vi "Initialize Run Files and Variables.vi"(0 "Start TIme X":refnum<vi>, 2 "System Idle Pressure X":refnum<vi>, 3 "Reactor Number":i32, 5 "Header Connection txt Array":refnum<vi>, 7 "Queue Reactor X":refnum<vi>, 8 "Stop / Start Reactor X":refnum<vi>, 9 "Reactor Name":string, 10 "Username X":refnum<vi>, 11 "Save File Connection X":refnum<vi>, 12 "Experimental Details X":refnum<vi>, 14 "ALD Sequence for Reactor X":refnum<vi>, 15 "Save File JSON Connection X":refnum<vi>, 16 "GUID X":refnum<vi>, 19 "Logging Data X":refnum<vi>) -> ()   [LabVIEW 2021]
uses:
  <vilib>/Utility/error.llb/DialogType.ctl
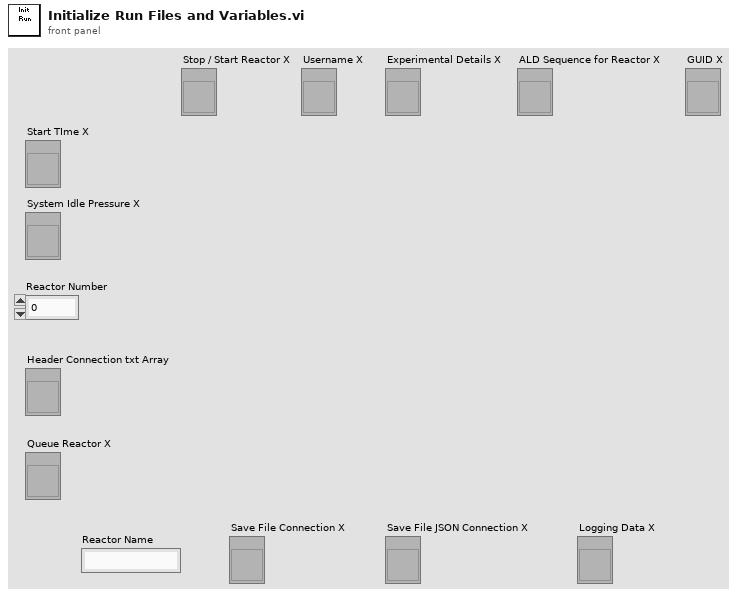
[diagram p1: front panel]
types:
  T1 = typedef "DialogType.ctl" = u16
  T2 = enum16{"open", "replace", "create", "open or create", "replace or create", "replace or create with confirmation"}
  T3 = cluster{"type":string, "meta":string, "payload":cluster{"GUID":string, "username":string, "experimentalDetails":string, "valveSequence":i32[][], "startTime":string, "reactorName":string}}
  T4 = cluster{"GUID":string, "username":string, "experimentalDetails":string, "valveSequence":i32[][], "startTime":string, "reactorName":string}
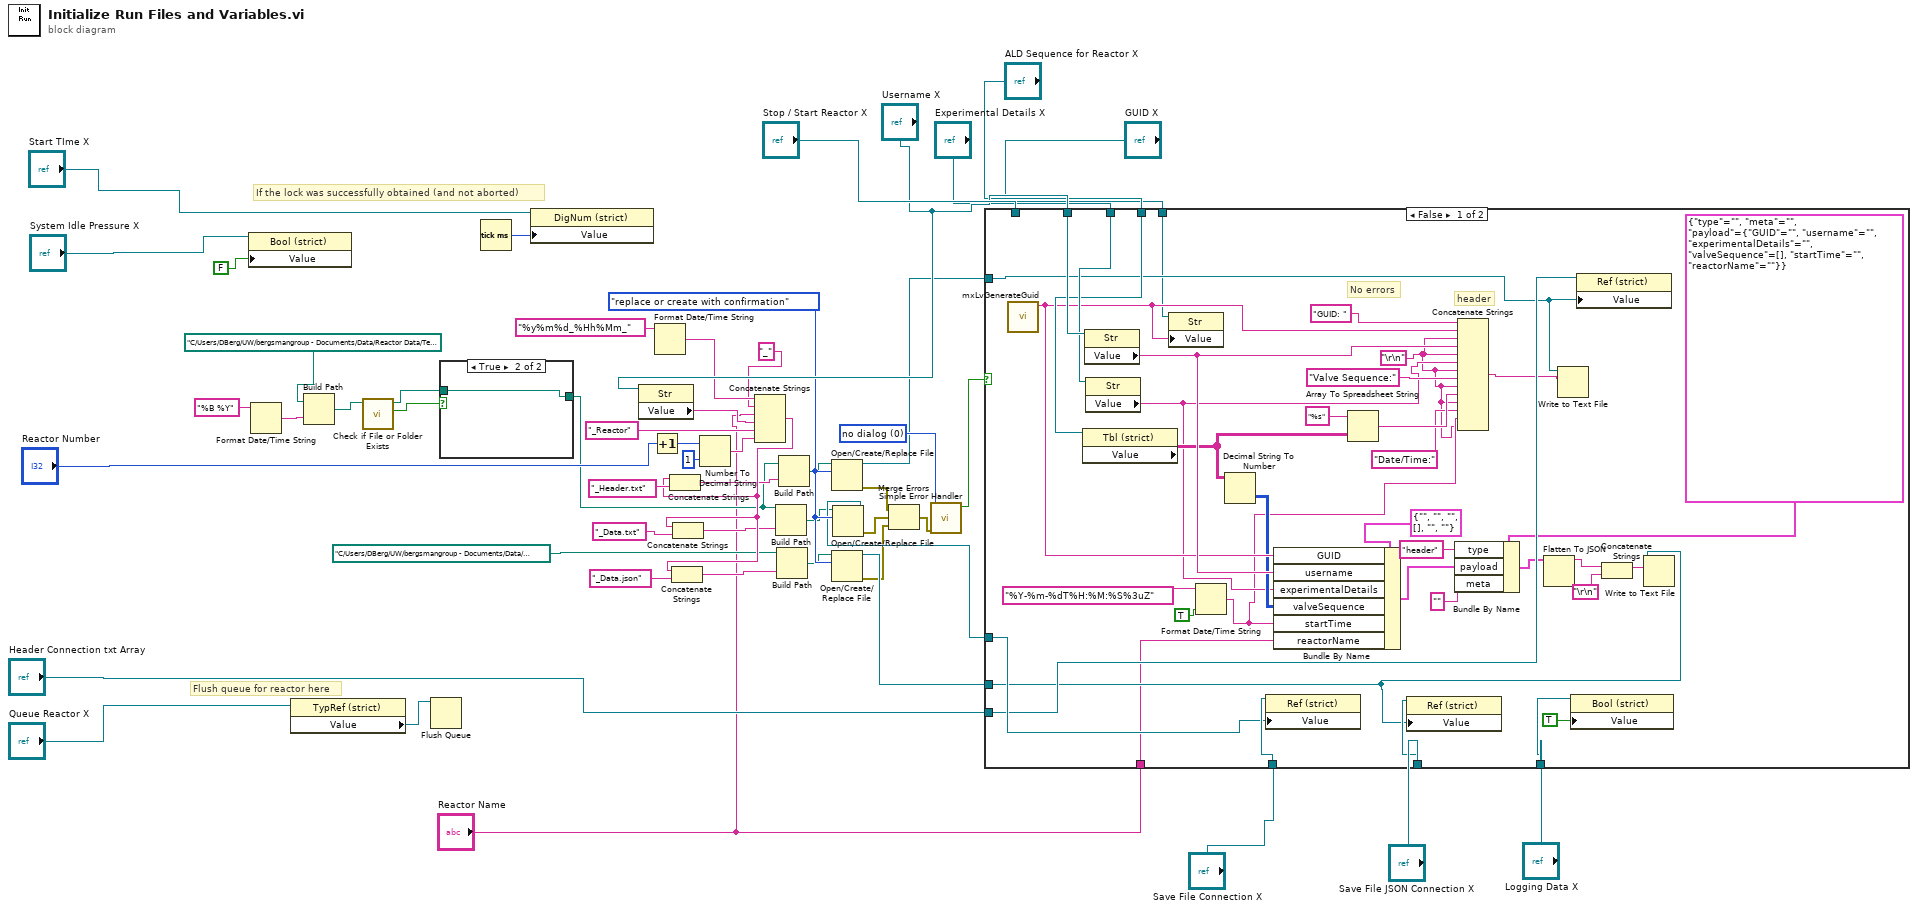
[diagram p0: block diagram]
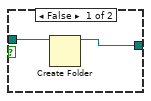
[diagram p2: hidden frame]
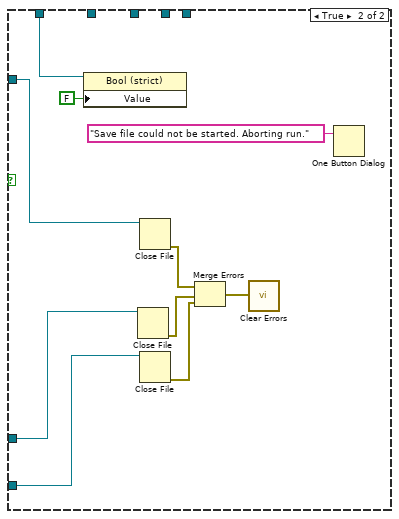
[diagram p3: hidden frame]
diagram:
  w31 = T1 0 items=["no dialog", "OK message", "continue or stop message", "OK message + warnings", "continue/stop + warnings"] ("type of dialog (OK msg:1)")
  w27 = T2."replace or create with confirmation" ("operation (0:open)")
  # "Flush queue for reactor here"
  # "If the lock was successfully obtained (and not aborted)"
  n1 = property class="Bool (strict)"(reference="System Idle Pressure X", "Value"=FALSE) -> ()  [unwired: 1 in, 2 out]
  n2 = Format Date/Time String(time format string (%c)="%B %Y") -> (date/time string=w9:string)  [unwired: 2 in]
  n3 = property class="TypRef (strict)"(reference="Queue Reactor X") -> ("Value"=w23:refnum<queue>)  [unwired: 1 in, 2 out]
  n4 = Build Path(base path=path "C:/Users/DBerg/UW/bergsmangroup - Documents/Data/Reactor Data/Text Files", name or relative path=w9) -> (appended path=w8:path)
  n5 = call <vilib>:"Check if File or Folder Exists.vi"("path"=w8) -> ("file or folder exists?"=w7:bool, "dup path"=w6:path)  [unwired: 8 in, 1 out]
  n6 = Flush Queue(queue=w23) -> ()  [unwired: 1 in, 3 out]
  n7 = case shown="True" w7 {
    tunnel: [w55 w56] -> w5
    tunnel: w6 -> [w54 w56]
    frame False {
      n8 = Create Folder(path (use dialog)=w54) -> (created path=w55:path)  [unwired: 2 in, 2 out]
    }
    frame True {
    }
  }
  n9 = Tick Count (ms)() -> (millisecond timer value=w36:u32)
  n10 = property class="DigNum (strict)"(reference="Start TIme X", "Value"=w36) -> ()  [unwired: 1 in, 2 out]
  n11 = property class="Str"(reference="Username X") -> ("Value"=w18:string)  [unwired: 1 in, 2 out]
  n12 = Increment(x="Reactor Number") -> (x+1=w37:i32)
  n13 = Format Date/Time String(time format string (%c)="%y%m%d_%Hh%Mm_") -> (date/time string=w3:string)  [unwired: 2 in]
  n14 = Number To Decimal String(number=w37, width (-)=i16 1) -> (decimal integer string=w19:string)
  n15 = Concatenate Strings(w3, "_" ("string"), "Reactor Name", w18, "_Reactor" ("string"), w19) -> (w29:string)
  n16 = Concatenate Strings(w29, "_Header.txt" ("string")) -> (w17:string)
  n17 = Concatenate Strings(w29, "_Data.json" ("string")) -> (w15:string)
  n18 = Concatenate Strings(w29, "_Data.txt" ("string")) -> (w16:string)
  n19 = Build Path(base path=w5, name or relative path=w16) -> (appended path=w13:path)
  n20 = Build Path(base path=path "C:/Users/DBerg/UW/bergsmangroup - Documents/Data/Reactor Data/JSON Files", name or relative path=w15) -> (appended path=w14:path)
  n21 = Build Path(base path=w5, name or relative path=w17) -> (appended path=w12:path)
  n22 = Open/Create/Replace File(file path (use dialog)=w12, operation (0:open)=w27) -> (refnum out=w25:refnum<file>, error out=w33:errorcluster)  [unwired: 4 in, 1 out]
  n23 = Open/Create/Replace File(file path (use dialog)=w14, operation (0:open)=w27) -> (refnum out=w24:refnum<file>, error out=w21:errorcluster)  [unwired: 4 in, 1 out]
  n24 = Open/Create/Replace File(file path (use dialog)=w13, operation (0:open)=w27) -> (refnum out=w26:refnum<file>, error out=w22:errorcluster)  [unwired: 4 in, 1 out]
  n25 = Merge Errors(w33, w22, w21) -> (w32:errorcluster)
  n26 = call <vilib>:"Simple Error Handler.vi"("type of dialog (OK msg:1)"=w31, "error in (no error)"=w32) -> ("error?"=w30:bool)  [unwired: 3 in, 4 out]
  n27 = case shown="False" w30 {
    tunnel: "Logging Data X" -> [w93 _]
    tunnel: "Stop / Start Reactor X" -> [_ w103]
    tunnel: "Username X" -> [w91 _]
    tunnel: "Experimental Details X" -> [w90 _]
    tunnel: "ALD Sequence for Reactor X" -> [w89 _]
    tunnel: "Save File Connection X" -> [w86 _]
    tunnel: w26 -> [w85 w99]
    tunnel: w25 -> [w80 w100]
    tunnel: "Save File JSON Connection X" -> [w83 _]
    tunnel: w24 -> [w72 w98]
    tunnel: "Header Connection txt Array" -> [w82 _]
    tunnel: "GUID X" -> [w78 _]
    tunnel: "Reactor Name" -> [w57 _]
    frame False {
      w66 = "\r\n"
      # "header"
      # "No errors"
      n28 = call <resource>:"mxLvGenerateGuid.vi"() -> ("Value"=w79:string)  [unwired: 10 in, 1 out]
      n29 = property class="Tbl (strict)"(reference=w89) -> ("Value"=w76:string[][])  [unwired: 1 in, 2 out]
      n30 = property class="Str"(reference=w91) -> ("Value"=w84:string)  [unwired: 1 in, 2 out]
      n31 = property class="Str"(reference=w90) -> ("Value"=w71:string)  [unwired: 1 in, 2 out]
      n32 = property class="Str"(reference=w78, "Value"=w79) -> ()  [unwired: 1 in, 2 out]
      n33 = Format Date/Time String(time format string (%c)="%Y-%m-%dT%H:%M:%S%3uZ", UTC format=TRUE) -> (date/time string=w67:string)  [unwired: 1 in]
      n34 = Decimal String To Number(string=w76) -> (number=w75:i32[][])  [unwired: 2 in, 1 out]
      n35 = property class="Ref (strict)"(reference=w86, "Value"=w85) -> ()  [unwired: 1 in, 2 out]
      n36 = Bundle By Name(cluster=T4 {"GUID"="", "username"="", "experimentalDetails"="", "valveSequence"=[], "startTime"="", "reactorName"=""}, "GUID"=w79, "username"=w84, "experimentalDetails"=w71, "valveSequence"=w75, "startTime"=w67, "reactorName"=w57) -> (w64:T4)
      n37 = Array To Spreadsheet String(array=w76, 3:"%s" ("format string")) -> (spreadsheet string=w77:string)  [unwired: 1 in]
      n38 = property class="Ref (strict)"(reference=w83, "Value"=w72) -> ()  [unwired: 1 in, 2 out]
      n39 = Bundle By Name(cluster=T3 {"type"="", "meta"="", "payload"={"GUID"="", "username"="", "experimentalDetails"="", "valveSequence"=[], "startTime"="", "reactorName"=""}} ("input cluster"), "type"="header", "payload"=w64, "meta"="") -> (w58:T3)
      n40 = Concatenate Strings("GUID: " ("string"), w79, w66, w84, w66, w71, w66, "Valve Sequence:" ("string"), w66, w77, w66, "Date/Time:" ("string"), w67, w66) -> (w81:string)
      n41 = Flatten To JSON(anything=w58) -> (JSON string=w59:string)  [unwired: 2 in, 1 out]
      n42 = Write to Text File(file (use dialog)=w80, text=w81) -> ()  [unwired: 2 in, 3 out]
      n43 = property class="Bool (strict)"(reference=w93, "Value"=TRUE) -> ()  [unwired: 1 in, 2 out]
      n44 = property class="Ref (strict)"(reference=w82, "Value"=w80) -> ()  [unwired: 1 in, 2 out]
      n45 = Concatenate Strings(w59, "\r\n") -> (w60:string)
      n46 = Write to Text File(file (use dialog)=w72, text=w60) -> ()  [unwired: 2 in, 3 out]
    }
    frame True {
      n47 = property class="Bool (strict)"(reference=w103, "Value"=FALSE) -> ()  [unwired: 1 in, 2 out]
      n48 = Close File(refnum=w99) -> (error out=w95:errorcluster)  [unwired: 1 in, 1 out]
      n49 = Close File(refnum=w100) -> (error out=w97:errorcluster)  [unwired: 1 in, 1 out]
      n50 = Close File(refnum=w98) -> (error out=w94:errorcluster)  [unwired: 1 in, 1 out]
      n51 = Merge Errors(w97, w95, w94) -> (w96:errorcluster)
      n52 = call <vilib>:"Clear Errors.vi"("error in (no error)"=w96) -> ()  [unwired: 5 in, 2 out]
      n53 = One Button Dialog(message="Save file could not be started. Aborting run.") -> ()  [unwired: 1 in, 1 out]
    }
  }
